vi "MoveIncMultiple.vi"(0 "controller in":refnum<k24>, 5 "axis names":string[](array[string]), 7 "speeds":dbl[](array[numeric]), 9 "distances":dbl[](array[numeric]), 11 "error in (no error)":errorcluster, 12 "return immediately":bool) -> (4 "controller out":refnum<k24>, 15 "error out":errorcluster)   [LabVIEW 2013]
uses:
  C:/GEECS/Developers Version/source/Device Driver/AerotechStage/Sample Vis/Bin/Aerotech.Ensemble.dll
  Bin/Aerotech.Ensemble.dll
  C:/GEECS/Developers Version/source/Device Driver/AerotechStage/Sample Vis/Bin/Aerotech.Ensemble.LabVIEW.dll
  Bin/Aerotech.Ensemble.LabVIEW.dll
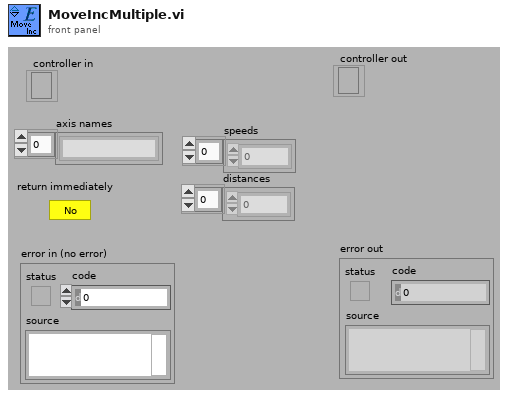
[diagram p1: front panel]
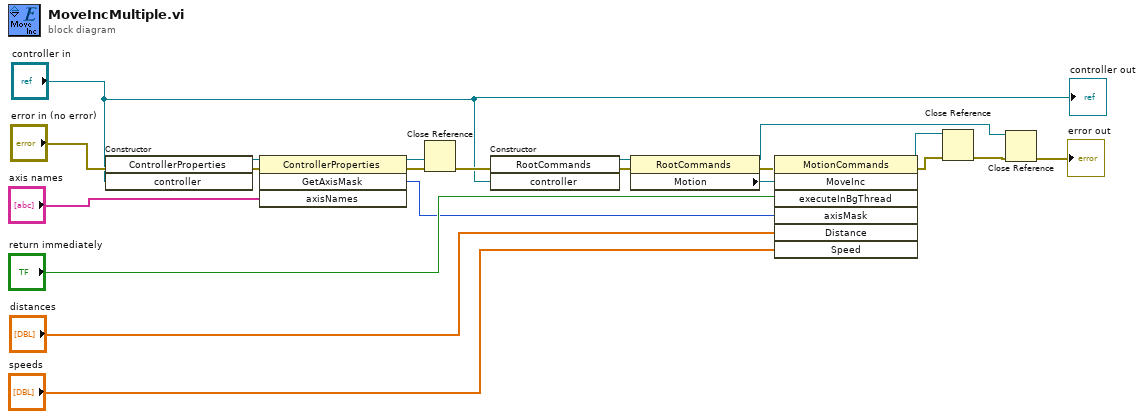
[diagram p0: block diagram]
diagram:
  n1 = constructor class="ControllerProperties"(error in="error in (no error)", "controller"="controller in") -> (reference out=w20:refnum<k24>, error out=w19:errorcluster)  [unwired: 2 in, 2 out]
  n2 = invoke class="ControllerProperties" method="GetAxisMask"(reference=w20, error in=w19, "axisNames"="axis names") -> (reference out=w17:refnum<k24>, error out=w18:errorcluster, "GetAxisMask"=w2:i32)  [unwired: 1 in, 1 out]
  n3 = Close Reference(reference=w17, error in (no error)=w18) -> (error out=w11:errorcluster)
  n4 = constructor class="RootCommands"(error in=w11, "controller"="controller in") -> (reference out=w8:refnum<k24>, error out=w7:errorcluster)  [unwired: 2 in, 2 out]
  n5 = property class="RootCommands"(reference=w8, error in=w7) -> (reference out=w3:refnum<k24>, error out=w9:errorcluster, "Motion"=w10:refnum<k24>)
  n6 = invoke class="MotionCommands" method="MoveInc"(reference=w10, error in=w9, "executeInBgThread"="return immediately", "axisMask"=w2, "Distance"="distances", "Speed"="speeds") -> (reference out=w5:refnum<k24>, error out=w6:errorcluster)  [unwired: 1 in, 5 out]
  n7 = Close Reference(reference=w5, error in (no error)=w6) -> (error out=w4:errorcluster)
  n8 = Close Reference(reference=w3, error in (no error)=w4) -> (error out=→"error out":errorcluster)
  "controller out" <- "controller in"
